vi "ECUMC 3 Selection Dialog.vi"(8 "error in (no error)":errorcluster, 9 "NIVS.System Definition Root":refnum<k24>, 11 "Links in":T1) -> (0 "error out":errorcluster, 3 "Links out":T1)   [LabVIEW 2011]
doc: "Use this template to create a dialog box with event handling."
uses:
  NationalInstruments.VeriStand.SystemStorage
  Controls/Control Links.ctl
  Controls/ECUMC Item.ctl
  <vilib>/ECUMC/NIVS/Support Files.llb/Item Type.ctl
  <vilib>/ECUMC/NIVS/Support Files.llb/XCP and CCP Master Custom Device.lvlib
panel:
  in  "ZMeas":bool
  in  "YMeas":bool
  in  "XMeas":bool
  in  "ZChar":bool
  in  "YChar":bool
  in  "XChar":bool
  out "Z Value":string
  out "Y Index":string
  out "X Index":string
  in  "Cancel":bool
  in  "Ok":bool
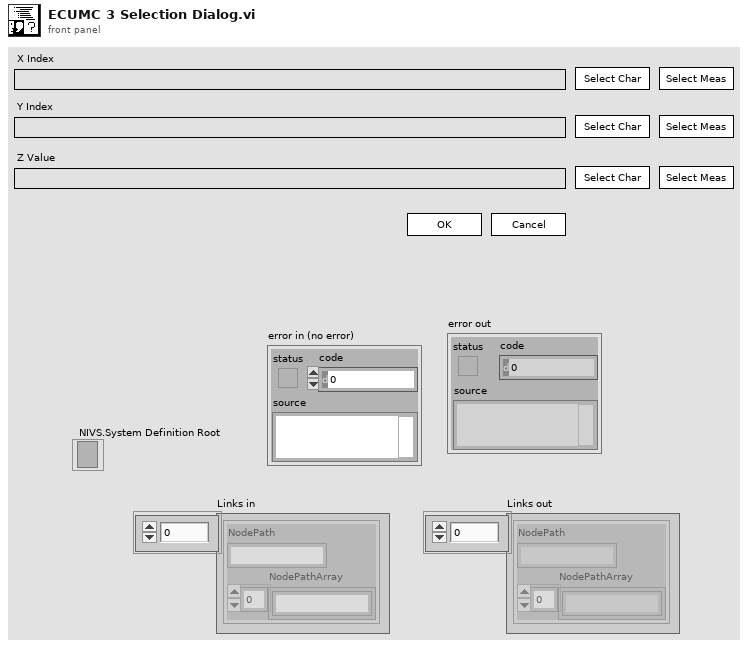
[diagram p1: front panel]
types:
  T1 = typedef "Control Links.ctl" = T2[]
  T2 = typedef "ECUMC Item.ctl" = cluster{"NodePath":string, "NodePathArray":string[]}
  T3 = typedef "XCP and CCP Master Custom Device.lvlib/Item Type.ctl" = enum16{"Scalar Characteristic", "Curve Characteristic", "Field Characteristic", "Measurement"}
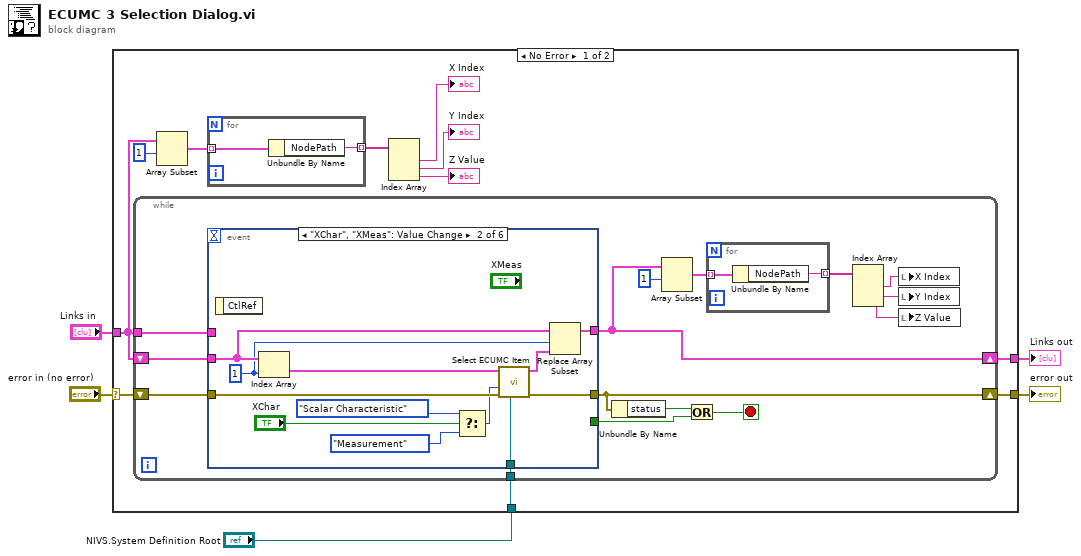
[diagram p0: block diagram]
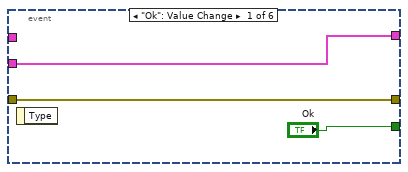
[diagram p2: hidden frame]
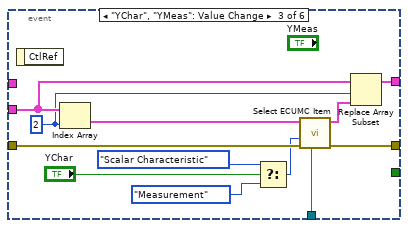
[diagram p3: hidden frame]
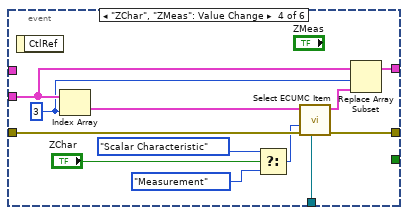
[diagram p4: hidden frame]
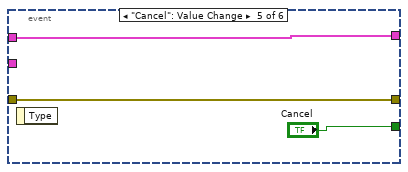
[diagram p5: hidden frame]
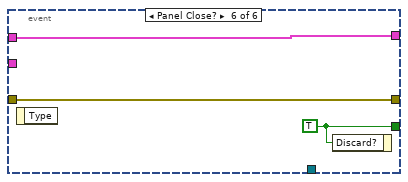
[diagram p6: hidden frame]
diagram:
  n1 = case shown="No Error" "error in (no error)" {
    selector: "error in (no error)" -> [w16 w82]
    tunnel: [w15 w82] -> w4
    tunnel: [w8 w81] -> w3
    tunnel: "Links in" -> [w7 w81]
    tunnel: "NIVS.System Definition Root" -> [w6 _]
    frame No Error {
      n2 = while {
        shift-right: [w29] -> w15
        shift-left: w16 -> [w30]
        shift-right: [w22] -> w8
        shift-left: w7 -> [w28]
        tunnel: w7 -> [w27]
        tunnel: w6 -> [w26]
        stop <- w32 stop-if-true
        n3 = event shown="[1] \"XChar\", \"XMeas\": Value Change" {
          selector: _ -> [_ _ _ _ _ _]
          dyn-events: _ -> [_ _ _ _ _ _]
          timeout: _ -> [_ _ _ _ _ _]
          tunnel: ["Ok" _ _ _ "Cancel" w80] -> w33
          tunnel: [w37 w49 w61 w73 w75 w79] -> w29
          tunnel: w30 -> [w37 w50 w62 w74 w75 w79]
          tunnel: w28 -> [w36 w46 w58 w70 _ _]
          tunnel: [w36 w45 w57 w69 w76 w78] -> w22
          tunnel: w27 -> [_ _ _ _ w76 w78]
          tunnel: w26 -> [_ w48 w60 w72 _ _]
          event "Ok": Value Change {
            n4 = event-data() -> ()  [unwired: 1 in, 1 out]
          }
          event "XChar", "XMeas": Value Change {
            w43 = 1 ("index")
            n5 = event-data() -> ()  [unwired: 1 in, 1 out]
            n6 = Index Array(array=w46, index=w43) -> (element=w47:T2)
            n7 = Select(t=Item_Type."Scalar Characteristic" ("Item Type"), s="XChar", f=Item_Type."Measurement" ("Item Type")) -> (s? t:f=w39:T3)
            n8 = call "Select ECUMC Item.vi"("NIVS.System Definition Root"=w48, "error in (no error)"=w50, "Item Type"=w39, "Link In"=w47) -> ("error out"=w49:errorcluster, "Link Out"=w44:T2)  [unwired: 5 in, 1 out]
            n9 = Replace Array Subset(array=w46, new element=w44, index=w43) -> (w45:T1)
          }
          event "YChar", "YMeas": Value Change {
            w55 = 2 ("index")
            n10 = event-data() -> ()  [unwired: 1 in, 1 out]
            n11 = Index Array(array=w58, index=w55) -> (element=w59:T2)
            n12 = Select(t=Item_Type."Scalar Characteristic" ("Item Type"), s="YChar", f=Item_Type."Measurement" ("Item Type")) -> (s? t:f=w52:T3)
            n13 = call "Select ECUMC Item.vi"("NIVS.System Definition Root"=w60, "error in (no error)"=w62, "Item Type"=w52, "Link In"=w59) -> ("error out"=w61:errorcluster, "Link Out"=w56:T2)  [unwired: 5 in, 1 out]
            n14 = Replace Array Subset(array=w58, new element=w56, index=w55) -> (w57:T1)
          }
          event "ZChar", "ZMeas": Value Change {
            w67 = 3 ("index")
            n15 = event-data() -> ()  [unwired: 1 in, 1 out]
            n16 = Index Array(array=w70, index=w67) -> (element=w71:T2)
            n17 = Select(t=Item_Type."Scalar Characteristic" ("Item Type"), s="ZChar", f=Item_Type."Measurement" ("Item Type")) -> (s? t:f=w64:T3)
            n18 = call "Select ECUMC Item.vi"("NIVS.System Definition Root"=w72, "error in (no error)"=w74, "Item Type"=w64, "Link In"=w71) -> ("error out"=w73:errorcluster, "Link Out"=w68:T2)  [unwired: 5 in, 1 out]
            n19 = Replace Array Subset(array=w70, new element=w68, index=w67) -> (w69:T1)
          }
          event "Cancel": Value Change {
            n20 = event-data() -> ()  [unwired: 1 in, 1 out]
          }
          event Panel Close? {
            w80 = TRUE ("Cancel")
            n21 = event-data() -> ()  [unwired: 1 in, 1 out]
            n22 = event-data("Discard?"=w80) -> ()  [unwired: 1 in, 1 out]
          }
        }
        n23 = Unbundle By Name(w29) -> ("status"=w31:bool)
        n24 = Array Subset(array=w22, index=1) -> (w24:T1)  [unwired: 1 in]
        n25 = Or(x=w31, y=w33) -> (x .or. y?=w32:bool)
        n26 = for {
          tunnel: w24 -> [w35] mode=indexing
          tunnel: [w34] -> w25 mode=indexing
          n27 = Unbundle By Name(w35) -> ("NodePath"=w34:string)
        }
        n28 = Index Array(array=w25) -> (element #1=w21:string, element #2=w20:string, element #3=w19:string)  [unwired: 3 in]
        n29 = local write "X Index"(w21) -> ()
        n30 = local write "Y Index"(w20) -> ()
        n31 = local write "Z Value"(w19) -> ()
      }
      n32 = Array Subset(array=w7, index=1) -> (w13:T1)  [unwired: 1 in]
      n33 = for {
        tunnel: w13 -> [w18] mode=indexing
        tunnel: [w17] -> w12 mode=indexing
        n34 = Unbundle By Name(w18) -> ("NodePath"=w17:string)
      }
      n35 = Index Array(array=w12) -> (element #1=→"X Index":string, element #2=→"Y Index":string, element #3=→"Z Value":string)  [unwired: 3 in]
    }
    frame Error {
    }
  }
  "error out" <- w4
  "Links out" <- w3
